vi "MT8852B Get Status if Needed.vi"(7 "Simulating? (F)":bool, 8 "error in (no error)":errorcluster, 11 "VISA session":refnum<visa-resource-name>) -> (0 "error out":errorcluster, 3 "VISA session out":refnum<visa-resource-name>)   [LabVIEW 2017]
doc: "Anritsu MT8850 Bluetooth Tester\n\nIf Instrument Status Checking is on, this VI will check the status byte and return an error if it is anything other than zero.\n\nINPUTS\n Simulating? - whether the instrument is in simulation mode or not."
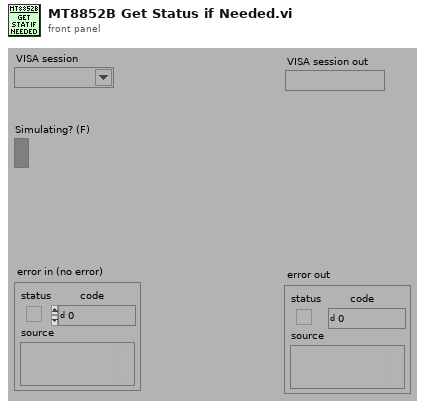
[diagram p1: front panel]
types:
  T1 = enum16{"Simulate", "Range check", "Cache", "Query instrument status"}
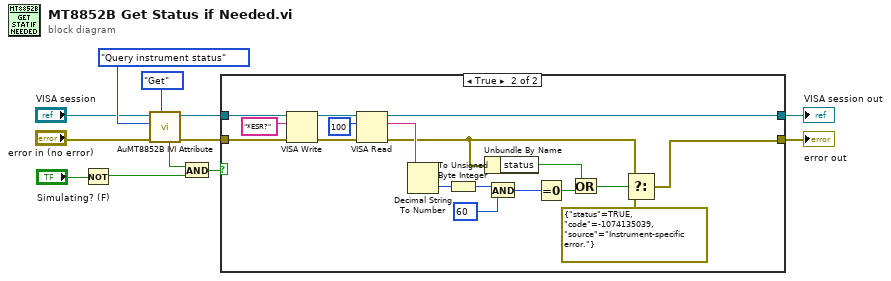
[diagram p0: block diagram]
diagram:
  n1 = Not(x="Simulating? (F)") -> (.not. x?=w2:bool)
  n2 = call <instrlib>:"AuMT8852B IVI Attribute.vi"("Set/Get (Set)"=enum16{"Set", "Get"}."Get", "error in (no error)"="error in (no error)", "Flag (Simulate)"=T1."Query instrument status", "VISA session"="VISA session") -> ("error out"=w9:errorcluster, "VISA session out"=w10:refnum<visa-resource-name>, "Value out"=w5:bool)  [unwired: 5 in]
  n3 = And(x=w5, y=w2) -> (x .and. y?=w6:bool)
  n4 = case shown="True" w6 {
    tunnel: w10 -> [w14 w32]
    tunnel: w9 -> [w13 w31]
    tunnel: [w13 w23] -> w8
    tunnel: [w14 w28] -> w7
    frame False {
    }
    frame True {
      n5 = VISA Write(VISA resource name=w32, write buffer="*ESR?" ("write buffer (\"\")"), error in (no error)=w31) -> (VISA resource name out=w30:refnum<visa-resource-name>, error out=w29:errorcluster)  [unwired: 1 out]
      n6 = VISA Read(VISA resource name=w30, byte count=u32 100 ("byte count (0)"), error in (no error)=w29) -> (VISA resource name out=w28:refnum<visa-resource-name>, read buffer=w25:string, error out=w18:errorcluster)  [unwired: 1 out]
      n7 = Decimal String To Number(string=w25) -> (number=w22:i32)  [unwired: 2 in, 1 out]
      n8 = To Unsigned Byte Integer(number=w22) -> (unsigned 8bit integer=w21:u8)
      n9 = Unbundle By Name(w18) -> ("status"=w16:bool)
      n10 = And(x=w21, y=u8 60) -> (x .and. y?=w19:u8)
      n11 = Equal To 0?(x=w19) -> (x = 0?=w17:bool)
      n12 = Or(x=w16, y=w17) -> (x .or. y?=w15:bool)
      n13 = Select(t=w18, s=w15, f=errorcluster {"status"=TRUE, "code"=-1074135039, "source"="Instrument-specific error."}) -> (s? t:f=w23:errorcluster)
    }
  }
  "error out" <- w8
  "VISA session out" <- w7
